vi "Distances from origin.vi"() -> ()   [LabVIEW 2020]
panel:
  in  "Template calibration":path=path "C:/Users/Dell/Documents/Vision-System/Images/calib-info.png"
  out "Array":string[](array[string])
  out "Image":T1(plugin-control)
  out "error out":errorcluster
  in  "error in (no error)":errorcluster
  in  "Image Path":path=path "C:/Users/Dell/Documents/Vision-System/Images/feltrino3.bmp"
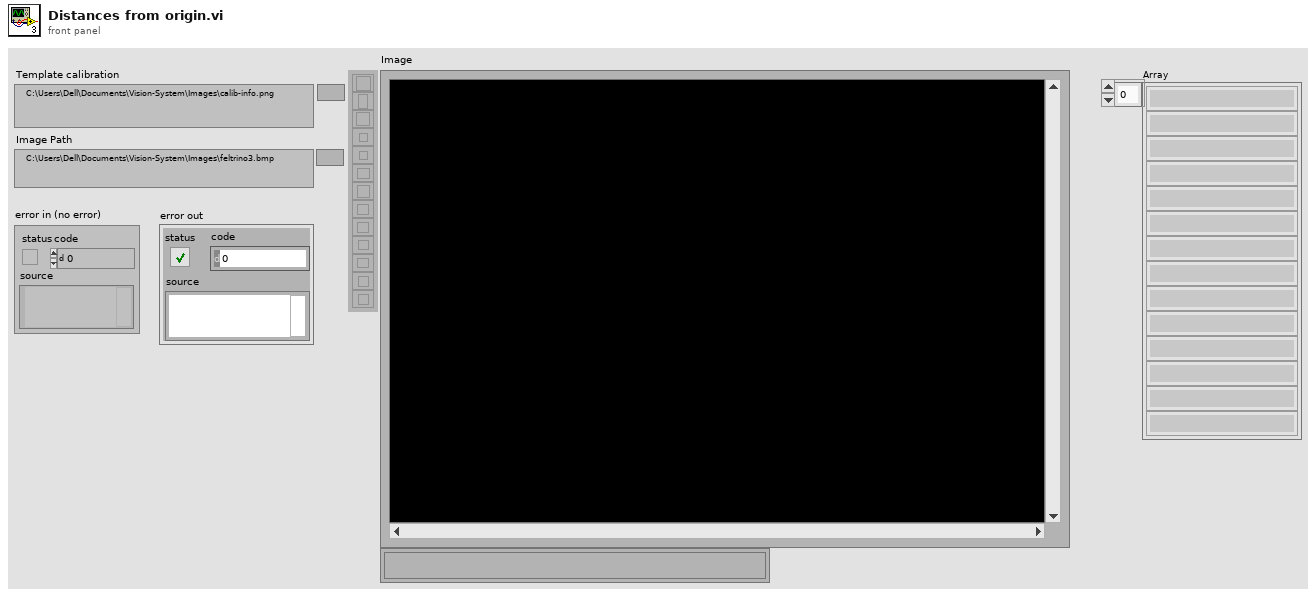
[diagram p1: front panel]
types:
  T1 = typedef "IMAQ Image.ctl" = refnum<image>
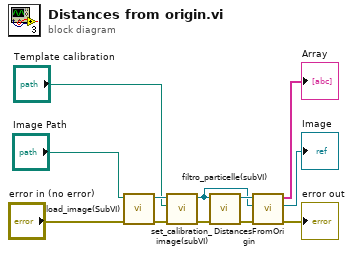
[diagram p0: block diagram]
diagram:
  n1 = call "load_image(SubVI).vi"("error in (no error)"="error in (no error)", "Image Path"="Image Path") -> ("error out"=w4:errorcluster, "Image GRAY"=w5:T1)  [unwired: 8 in]
  n2 = call "set_calibration_image(subVI).vi"("error in (no error)"=w4, "File Path"="Template calibration", "Image Dst"=w5) -> ("error out"=w6:errorcluster, "Image Out"=w1:T1)  [unwired: 6 in, 1 out]
  n3 = call "filtro_particelle(subVI).vi"("error in (no error)"=w6, "Image Src"=w1) -> ("error out"=w12:errorcluster, "Image"=w8:T1)  [unwired: 8 in]
  n4 = call "DistancesFromOrigin.vi"("error in (no error)"=w12, "Image Dst"=w1, "Image Src"=w8) -> ("error out"=→"error out":errorcluster, "Image Out"=→"Image":T1, "Array"=→"Array":string[])  [unwired: 6 in]
